vi "crashdetect.vi"   [LabVIEW 2015]
doc: "Update global variable indicating whether the aircraft has crashed.\nThe aircraft is determined to have crashed if it exceed 5g gravity at any time."
uses:
  global.vi
types:
  T1 = cluster{"Airspeed":dbl, "Altitude":dbl, "Vertical Speed":dbl, "Pitch":dbl, "Roll":dbl, "Heading":dbl, "Turn Indicator":dbl, "Latitude":dbl, "Longitude":dbl, "pilot g":dbl, "view number":i16, "fov":dbl, "view heading":dbl, "view pitch":dbl, "game width":i16, "game height":i16}
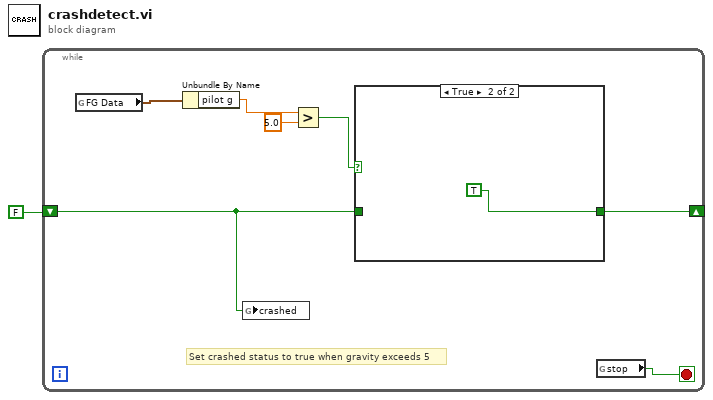
[diagram p0: block diagram]
diagram:
  n1 = while {
    shift-right: [w4] -> _
    shift-left: FALSE -> [w3]
    stop <- w2 stop-if-true
    # "Set crashed status to true when gravity exceeds 5"
    n2 = global read "global.vi" "FG Data"() -> (w8:T1)
    n3 = Unbundle By Name(w8) -> ("pilot g"=w7:dbl)
    n4 = global write "global.vi" "crashed"(w3) -> ()
    n5 = Greater?(x=w7, y=5.0) -> (0:w5:bool)
    n6 = case shown="True" w5 {
      tunnel: w3 -> [w9 _]
      tunnel: [w9 TRUE] -> w4
      frame False {
      }
      frame True {
      }
    }
    n7 = global read "global.vi" "stop"() -> (w2:bool)
  }
